vi "WidebandDecompose.vi"(4 "high cutoff freq: fh":dbl=100.0 format="%#_13g", 6 "low cutoff freq: fl":dbl=30.0 format="%#_13g", 9 "Spike Threshold":dbl format="%0.2f", 10 "dt":dbl, 11 "input wave":dbl[](array[numeric])) -> (0 "Gamma Wave":waveform(dbl), 1 "spiking":waveform(i16), 2 "lfp":waveform(dbl), 3 "mu":waveform(dbl))   [LabVIEW 2014]
uses:
  <vilib>/Analysis/3filter.llb/Filter Passband Type.ctl
  <vilib>/Analysis/3filter.llb/Butterworth Filter (DBL).vi
  <vilib>/ptbypt/NI_PtbyPt.lvlib
  <vilib>/Analysis/NI_AALBase.lvlib
types:
  T1 = typedef "NI_AALBase.lvlib/Filter Passband Type.ctl" = enum32{"Lowpass", "Highpass", "Bandpass", "Bandstop"}
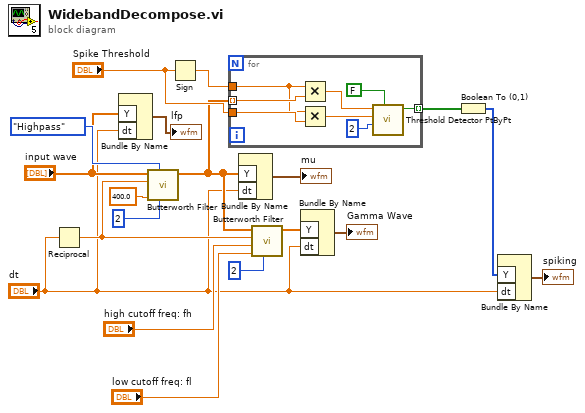
[diagram p0: block diagram]
diagram:
  n1 = Reciprocal(x="dt") -> (1/x=w7:dbl)
  n2 = Bundle By Name("Y"="input wave", "dt"="dt") -> (→"lfp":waveform(dbl))  [unwired: 1 in]
  n3 = call-poly <vilib>:"Butterworth Filter.vi"("order"=2, "filter type"=Filter_Passband_Type."Highpass", "low cutoff freq: fl"=400.0, "sampling freq: fs"=w7, "X"="input wave") -> ("Filtered X"=w8:dbl[])  [unwired: 3 in, 1 out]
  n4 = Sign(1:"Spike Threshold") -> (0:w10:dbl)
  n5 = for {
    tunnel: w8 -> [w24] mode=indexing
    tunnel: "Spike Threshold" -> [w22]
    tunnel: [w25] -> w16 mode=indexing
    tunnel: w10 -> [w21]
    n6 = Multiply(x=w21, y=w24) -> (x*y=w23:dbl)
    n7 = Multiply(x=w21, y=w22) -> (x*y=w20:dbl)
    n8 = call <vilib>:"Threshold Detector PtByPt.vi"("initialize"=FALSE, "width"=2, "threshold"=w20, "x"=w23) -> ("detected"=w25:bool)  [unwired: 5 in, 2 out]
  }
  n9 = Bundle By Name("Y"=w8, "dt"="dt") -> (→"mu":waveform(dbl))  [unwired: 1 in]
  n10 = call-poly <vilib>:"Butterworth Filter.vi"("order"=2, "low cutoff freq: fl"="low cutoff freq: fl", "high cutoff freq: fh"="high cutoff freq: fh", "sampling freq: fs"=w7, "X"=w8) -> ("Filtered X"=w4:dbl[])  [unwired: 3 in, 1 out]
  n11 = Bundle By Name("Y"=w4, "dt"="dt") -> (→"Gamma Wave":waveform(dbl))  [unwired: 1 in]
  n12 = Boolean To (0,1)(Boolean=w16) -> (0, 1=w15:i16[])
  n13 = Bundle By Name("Y"=w15, "dt"="dt") -> (→"spiking":waveform(i16))  [unwired: 1 in]
